vi "Add Dirty Dot.vi"(8 "error in (no error)":errorcluster, 11 "Cfg Grandmaster in":refnum<class "Cfg Grandmaster.lvclass">) -> (0 "error out":errorcluster, 1 "Canceled?":bool, 3 "Cfg Grandmaster out":refnum<class "Cfg Grandmaster.lvclass">)   [LabVIEW 2018, in "Configuration Grandmaster.lvlib" / "Cfg Grandmaster.lvclass"]
uses:
  Cfg Grandmaster.lvclass
  Cfg Grandmaster.lvclass/Cfg Grandmaster.ctl
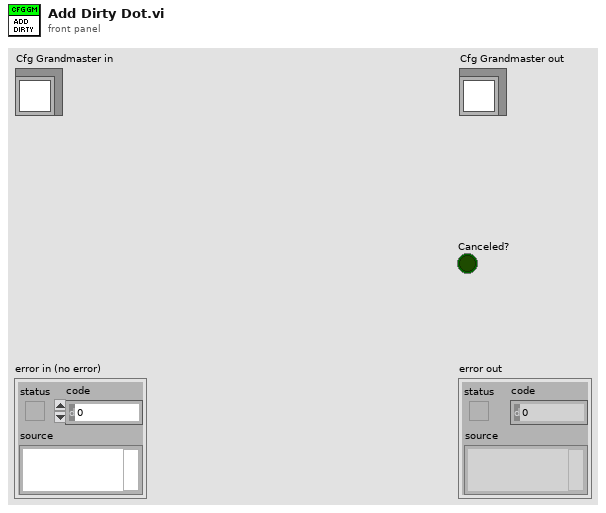
[diagram p1: front panel]
types:
  T1 = typedef "ge_Cfg wChassis.ctl" = cluster{"Chassis BOM":refnum<class "Chassis BOM.lvclass">, "Chassis Cfg":refnum<class "ChassisCfg.lvclass">, "Chassis Tasks":refnum<class "Chassis Tasks.lvclass">, "HW Error":bool, "Unsvd Chgs?":bool}
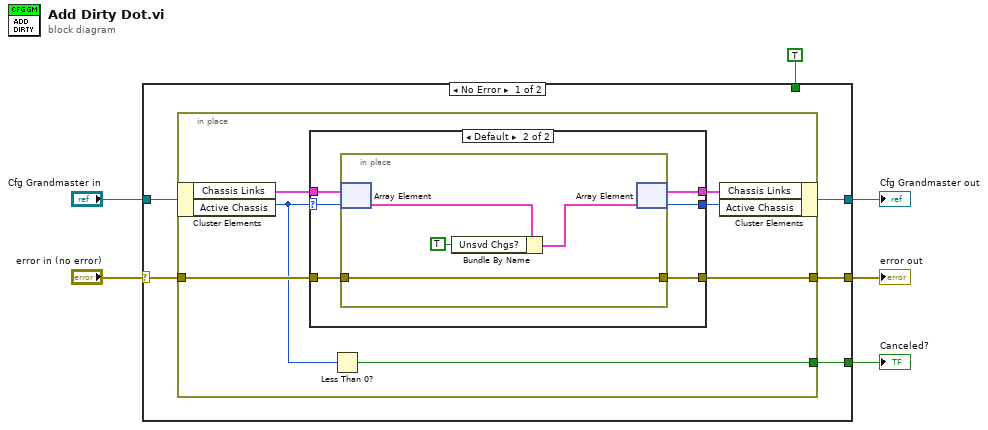
[diagram p0: block diagram]
diagram:
  n1 = case shown="No Error" "error in (no error)" {
    selector: "error in (no error)" -> [w10 w34]
    tunnel: [w11 w34] -> w5
    tunnel: [w8 w33] -> w3
    tunnel: "Cfg Grandmaster in" -> [w9 w33]
    tunnel: [w7 w32] -> w2
    tunnel: TRUE -> [_ w32]
    frame No Error {
      n2 = in-place {
        in-place-border: [w18] -> w11
        in-place-border: w10 -> [w17]
        in-place-border: [w12] -> w7
        n3 = in-place-cluster #1(w9) -> ("Chassis Links"=w16:T1[], "Active Chassis"=w15:i32)
        n4 = case shown="Default" w15 {
          selector: w15 -> [w19 w23]
          tunnel: w17 -> [w20 w27]
          tunnel: [w20 w26] -> w18
          tunnel: w16 -> [w21 w25]
          tunnel: [w21 w24] -> w13
          tunnel: [w19 w22] -> w14
          frame -1 {
          }
          frame Default {
            n5 = in-place {
              in-place-border: w27 -> [w28]
              in-place-border: [w28] -> w26
              n6 = in-place-array #2(w25, w23) -> (w31:T1)
              n7 = Bundle By Name(cluster=w31, "Unsvd Chgs?"=TRUE) -> (w30:T1)
              n8 = in-place-array #2(w30) -> (w24:T1[], w22:i32)
            }
          }
        }
        n9 = Less Than 0?(x=w15) -> (x < 0?=w12:bool)
        n10 = in-place-cluster #1("Chassis Links"=w13, "Active Chassis"=w14) -> (w8:refnum<class "Cfg Grandmaster.lvclass">)
      }
    }
    frame Error {
    }
  }
  "error out" <- w5
  "Cfg Grandmaster out" <- w3
  "Canceled?" <- w2
